vi "4.vi"() -> ()   [LabVIEW 2017, in "ErrorStructureDrawer-Tests.lvlib"]
uses:
  ErrorStructureDrawer-Tests.lvlib
panel:
  out "Numeric 2":i32
  out "Numeric":i32
  in  "Array 2":i32[](array[numeric])
  in  "Array":i32[](array[numeric])
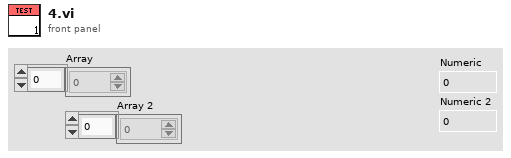
[diagram p1: front panel]
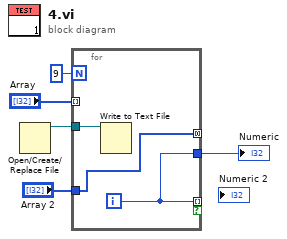
[diagram p0: block diagram]
diagram:
  n1 = Open/Create/Replace File() -> (refnum out=w1:refnum<file>)  [unwired: 6 in, 2 out]
  n2 = for {
    N: 9 -> [_]
    tunnel: w1 -> [w8]
    tunnel: [w7] -> _ mode=indexing if=_
    tunnel: "Array" -> [_] mode=indexing
    tunnel: "Array 2" -> [w6]
    tunnel: [w7] -> w3
    tunnel: [w6] -> _ mode=concatenating
    i -> [w7]
    n3 = Write to Text File(file (use dialog)=w8) -> ()  [unwired: 3 in, 3 out]
  }
  "Numeric" <- w3
